vi "Get LakeShore 370 Resistance_VISA.vi"(4 "Read channel":enum16{"Default (1)", "Latest scan selection"}(ring)=enum."Latest scan selection", 6 "Read temperature":bool, 7 "Read heater":bool, 8 "error in (no error)":errorcluster, 9 "Seconds between samples":dbl=1.0 format="%_4f", 10 "Channels to scan (empty = don't use scanner option)":i32[](array[numeric]), 11 "VISA resource name":refnum<visa-resource-name>) -> (0 "error out":errorcluster, 2 "Resistance":dbl[](array[numeric]) format="%#_6p", 3 "VISA resource name out":refnum<visa-resource-name>)   [LabVIEW 2021]
uses:
  GPIB/VISA  Send Receive.vi
  Simple VISA Reader/Simple VISA Reader Driver.lvclass
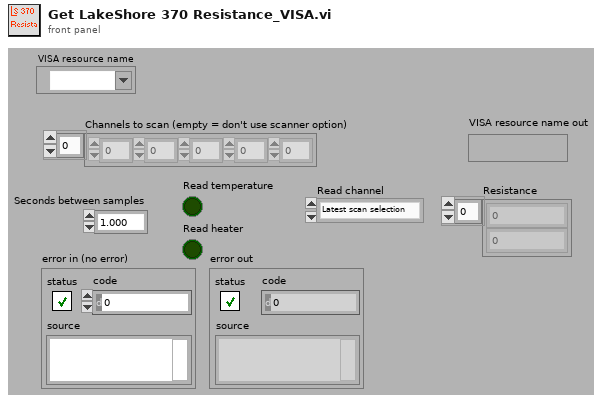
[diagram p1: front panel]
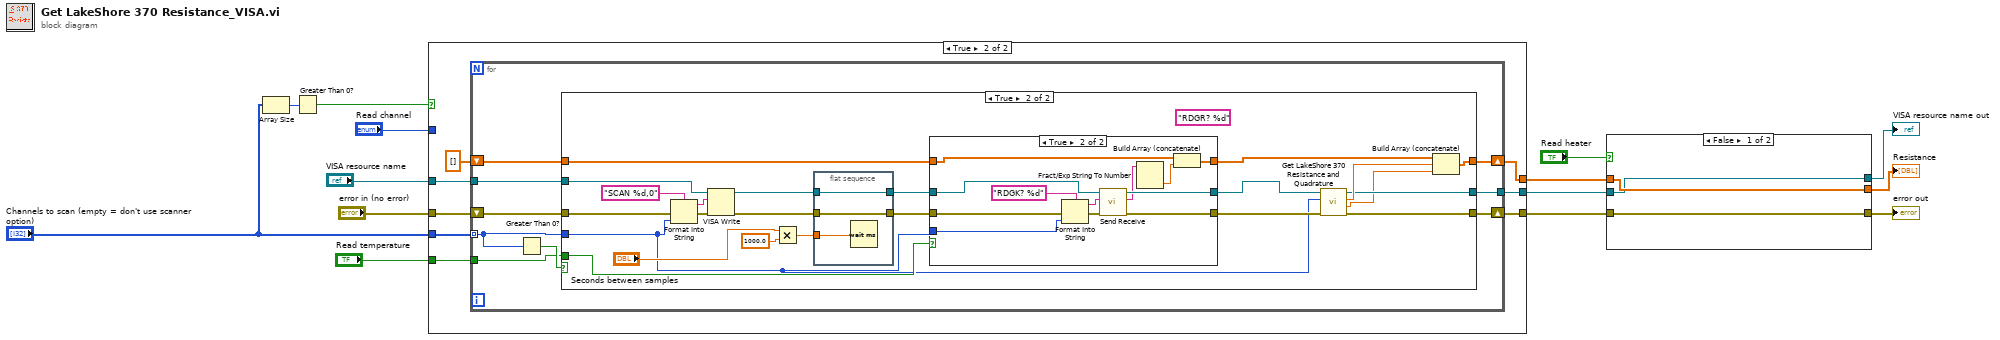
[diagram p0: block diagram]
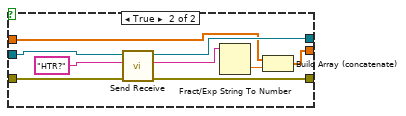
[diagram p2: hidden frame]
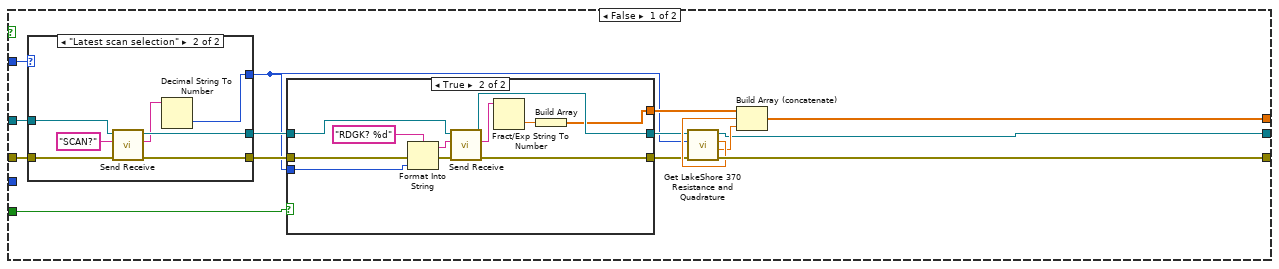
[diagram p3: hidden frame]
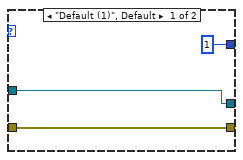
[diagram p4: hidden frame]
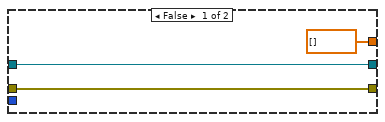
[diagram p5: hidden frame]
diagram:
  n1 = Array Size(array="Channels to scan (empty = don't use scanner option)") -> (size(s)=w14:i32)
  n2 = Greater Than 0?(x=w14) -> (x > 0?=w13:bool)
  n3 = case shown="True" w13 {
    tunnel: "Channels to scan (empty = don't use scanner option)" -> [_ w61]
    tunnel: [w29 w60] -> w4
    tunnel: "error in (no error)" -> [w26 w59]
    tunnel: [w21 w58] -> w8
    tunnel: "VISA resource name" -> [w25 w56]
    tunnel: [w18 w55] -> w6
    tunnel: "Read temperature" -> [w28 w54]
    tunnel: "Read channel" -> [w22 _]
    frame False {
      n4 = case shown="\"Latest scan selection\"" w22 {
        tunnel: w26 -> [w32 w39]
        tunnel: [w32 w38] -> w23
        tunnel: w25 -> [w31 w36]
        tunnel: [w31 w35] -> w24
        tunnel: [1 w33] -> w15
        frame "Default (1)", Default {
        }
        frame "Latest scan selection" {
          n5 = call-poly "Send Receive.vi"("error in (no error)"=w39, "data string in"="SCAN?", "VISA Resource Name"=w36) -> ("error out"=w38:errorcluster, "data string out"=w34:string, "VISA Resource Name Out"=w35:refnum<visa-resource-name>)  [unwired: 6 in]
          n6 = Decimal String To Number(string=w34) -> (number=w33:i32)  [unwired: 2 in, 1 out]
        }
      }
      n7 = case shown="True" w28 {
        tunnel: w23 -> [w42 w47]
        tunnel: [w42 w53] -> w16
        tunnel: w24 -> [w41 w52]
        tunnel: [w41 w51] -> w17
        tunnel: [dbl[] [] w48] -> w27
        tunnel: w15 -> [_ w43]
        frame False {
        }
        frame True {
          n8 = Format Into String(format string="RDGK? %d" ("data string in"), error in=w47, w43) -> (resulting string=w44:string, error out=w46:errorcluster)  [unwired: 1 in]
          n9 = call-poly "Send Receive.vi"("error in (no error)"=w46, "data string in"=w44, "VISA Resource Name"=w52) -> ("error out"=w53:errorcluster, "data string out"=w50:string, "VISA Resource Name Out"=w51:refnum<visa-resource-name>)  [unwired: 6 in]
          n10 = Fract/Exp String To Number(string=w50) -> (number=w49:dbl)  [unwired: 4 out]
          n11 = Build Array(w49) -> (w48:dbl[])
        }
      }
      n12 = call "Get LakeShore 370 Resistance and Quadrature.vi"("error in"=w16, "Channel"=w15, "VISA resource name"=w17) -> ("error out"=w21:errorcluster, "Q"=w19:dbl, "R"=w20:dbl, "VISA resource name out"=w18:refnum<visa-resource-name>)  [unwired: 5 in]
      n13 = Build Array (concatenate)(w27, w20, w19) -> (w29:dbl[])
    }
    frame True {
      n14 = for {
        tunnel: w61 -> [w64] mode=indexing
        shift-right: [w67] -> w60
        shift-left: dbl[] [] -> [w66]
        shift-right: [w68] -> w58
        shift-left: w59 -> [w70]
        tunnel: w56 -> [w65]
        tunnel: [w63] -> w55
        tunnel: w54 -> [w62]
        n15 = Greater Than 0?(x=w64) -> (x > 0?=w69:bool)
        n16 = case shown="True" w69 {
          tunnel: w64 -> [_ w75]
          tunnel: w70 -> [w72 w86]
          tunnel: [w72 w89] -> w68
          tunnel: [w73 w93] -> w67
          tunnel: w66 -> [w73 w77]
          tunnel: w65 -> [w71 w88]
          tunnel: [w71 w83] -> w63
          tunnel: w62 -> [_ w78]
          frame False {
          }
          frame True {
            (unwired) "RDGR? %d" ("data string in")
            n17 = Format Into String(format string="SCAN %d,0", error in=w86, w75) -> (resulting string=w87:string, error out=w85:errorcluster)  [unwired: 1 in]
            n18 = VISA Write(VISA resource name=w88, write buffer=w87, error in (no error)=w85) -> (VISA resource name out=w84:refnum<visa-resource-name>, error out=w91:errorcluster)  [unwired: 1 out]
            n19 = Multiply(x="Seconds between samples", y=1000.0) -> (x*y=w94:dbl)
            n20 = flat-sequence {
              tunnel: [w113] -> w82
              tunnel: w94 -> [w114]
              tunnel: w91 -> [w113]
              tunnel: w84 -> [w112]
              tunnel: [w112] -> w80
              frame #0 {
                n21 = Wait (ms)(milliseconds to wait=w114) -> ()  [unwired: 1 out]
              }
            }
            n22 = case shown="True" w78 {
              tunnel: w82 -> [w99 w104]
              tunnel: [w99 w111] -> w81
              tunnel: w80 -> [w98 w110]
              tunnel: [w98 w109] -> w79
              tunnel: w77 -> [w97 w107]
              tunnel: [w97 w105] -> w76
              tunnel: w75 -> [_ w101]
              frame False {
              }
              frame True {
                n23 = Format Into String(format string="RDGK? %d" ("data string in"), error in=w104, w101) -> (resulting string=w100:string, error out=w103:errorcluster)  [unwired: 1 in]
                n24 = call-poly "Send Receive.vi"("error in (no error)"=w103, "data string in"=w100, "VISA Resource Name"=w110) -> ("error out"=w111:errorcluster, "data string out"=w108:string, "VISA Resource Name Out"=w109:refnum<visa-resource-name>)  [unwired: 6 in]
                n25 = Fract/Exp String To Number(string=w108) -> (number=w106:dbl)  [unwired: 4 out]
                n26 = Build Array (concatenate)(w107, w106) -> (w105:dbl[])
              }
            }
            n27 = call "Get LakeShore 370 Resistance and Quadrature.vi"("error in"=w81, "Channel"=w75, "VISA resource name"=w79) -> ("error out"=w89:errorcluster, "Q"=w74:dbl, "R"=w90:dbl, "VISA resource name out"=w83:refnum<visa-resource-name>)  [unwired: 5 in]
            n28 = Build Array (concatenate)(w76, w90, w74) -> (w93:dbl[])
          }
        }
      }
    }
  }
  n29 = case shown="False" "Read heater" {
    tunnel: w8 -> [w116 w126]
    tunnel: [w116 w125] -> w7
    tunnel: w6 -> [w115 w124]
    tunnel: [w115 w123] -> w5
    tunnel: w4 -> [w117 w121]
    tunnel: [w117 w119] -> w3
    frame False {
    }
    frame True {
      n30 = call-poly "Send Receive.vi"("error in (no error)"=w126, "data string in"="HTR?", "VISA Resource Name"=w124) -> ("error out"=w125:errorcluster, "data string out"=w122:string, "VISA Resource Name Out"=w123:refnum<visa-resource-name>)  [unwired: 6 in]
      n31 = Fract/Exp String To Number(string=w122) -> (number=w120:dbl)  [unwired: 4 out]
      n32 = Build Array (concatenate)(w121, w120) -> (w119:dbl[])
    }
  }
  "error out" <- w7
  "Resistance" <- w3
  "VISA resource name out" <- w5
